vi "Set Legend (WFChart).vi"(8 "error in (no error)":errorcluster, 10 "Plot.Plot Name":string[](array[string]), 11 "WaveformChart in":refnum<vi>) -> (0 "error out":errorcluster)   [LabVIEW 2019, in "Instrument.Lockin.lvlib" / "Instrument UI.Lockin.lvclass"]
uses:
  Instrument UI.Lockin.lvclass
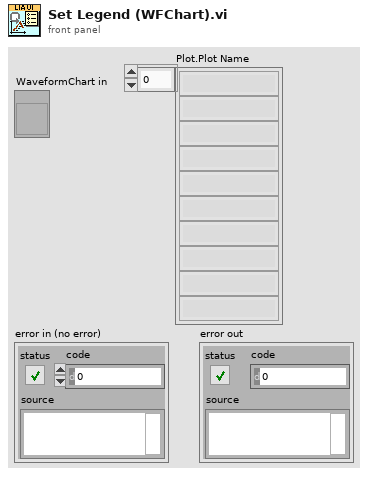
[diagram p1: front panel]
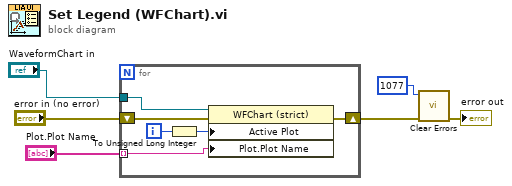
[diagram p0: block diagram]
diagram:
  n1 = for {
    tunnel: "Plot.Plot Name" -> [w11] mode=indexing
    shift-right: [w12] -> w5
    shift-left: "error in (no error)" -> [w8]
    tunnel: "WaveformChart in" -> [w9]
    i -> [w7]
    n2 = To Unsigned Long Integer(number=w7) -> (unsigned 32bit integer=w10:u32)
    n3 = property on="Property Node" class="WFChart (strict)"(reference=w9, error in=w8, "Active Plot"=w10, "Plot.Plot Name"=w11) -> (error out=w12:errorcluster)  [unwired: 1 out]
  }
  n4 = call <vilib>:"Clear Errors.vi"("error in (no error)"=w5, "specific error code to clear (0: all)"=1077) -> ("error out"=→"error out":errorcluster)  [unwired: 4 in, 1 out]
